vi "Configure Bandwidth Limit.vi"(8 "error in (no error)":errorcluster, 9 "Bandwidth Limit (0: 20MHz)":i32(ring) items=["20MHz", "200MHz", "1.5GHz", "3GHz", "25MHz"], 10 "Channel (1: Channel 1)":i32(ring)=1 items=["Channel 1"=1, "Channel 2"=2, "Channel 3"=3, "Channel 4"=4], 11 "VISA resource name":refnum<visa-resource-name>) -> (0 "error out":errorcluster, 3 "VISA resource name out":refnum<visa-resource-name>)   [LabVIEW 2017, in "Agilent 2000 3000 X-Series.lvlib"]
doc: "Sets the bandwidth limit value and enables bandwidth limiting for the selected channel. Use the <b>Configure Channel Characteristics</b> VI to disable bandwidth limiting and the <b>Configure Channel</b> VI to configure other settings for the channel including input impedance.\n\n<b>Note:</b>\nThis VI is specific to the 6000-X Series oscilloscopes. These features are not available on other models."
uses:
  Agilent 2000 3000 X-Series.lvlib
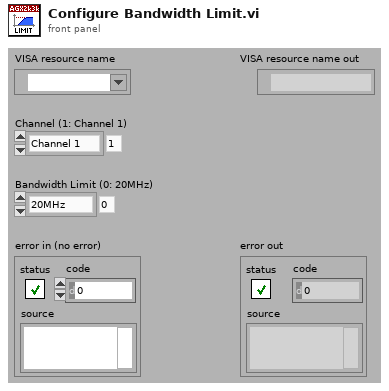
[diagram p1: front panel]
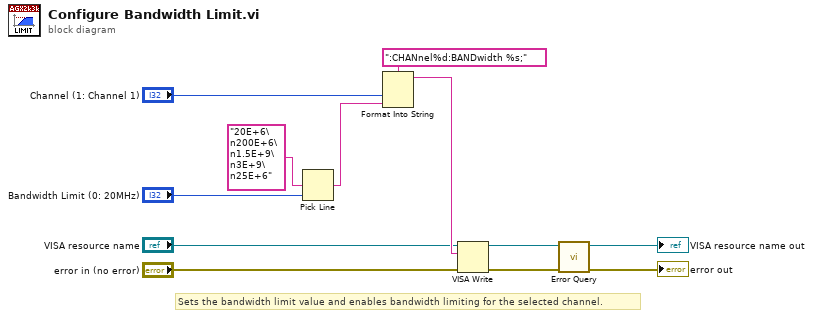
[diagram p0: block diagram]
diagram:
  # "Sets the bandwidth limit value and enables bandwidth limiting for the selected channel."
  n1 = Pick Line(multi-line string="20E+6\n200E+6\n1.5E+9\n3E+9\n25E+6", line index="Bandwidth Limit (0: 20MHz)") -> (output string=w6:string)  [unwired: 1 in]
  n2 = Format Into String(format string=":CHANnel%d:BANDwidth %s;", "Channel (1: Channel 1)", w6) -> (resulting string=w10:string)  [unwired: 2 in, 1 out]
  n3 = VISA Write(VISA resource name="VISA resource name", write buffer=w10, error in (no error)="error in (no error)") -> (VISA resource name out=w4:refnum<visa-resource-name>, error out=w3:errorcluster)  [unwired: 1 out]
  n4 = call "Error Query.vi"("error in (no error)"=w3, "VISA resource name"=w4) -> ("error out"=→"error out":errorcluster, "VISA resource name out"=→"VISA resource name out":refnum<visa-resource-name>)  [unwired: 6 in, 2 out]
